vi "Main.vi"() -> ()   [LabVIEW 2014, in "Step Genie.lvlib"]
uses:
  Step Genie.lvlib
  <vilib>/Utility/error.llb/DialogType.ctl
  Source/SLL Queued State Machine/Queue Driver/Create Queue.vi
  Source/SLL Queued State Machine/Queue Driver/Enqueue an Item to Queue.vi
  Source/SLL Queued State Machine/Queue Driver/Dequeue Queue.vi
  Source/SLL Queued State Machine/Queue Driver/Enqueue N Items.vi
  Source/SLL Queued State Machine/Queue Driver/Flush Queue.vi
  Source/SLL Queued State Machine/Queue Driver/Release Queue.vi
  Source/SLL Queued State Machine/SLL QSM.lvlib
  Source/SLL Spreadsheet/SLL Spreadsheet.lvlib
panel:
  in  "Title":string(combo)
  in  "Fail":bool
  in  "Skip":bool
  in  "Pass":bool
  in  "Comments":string
  out "Instructions":string
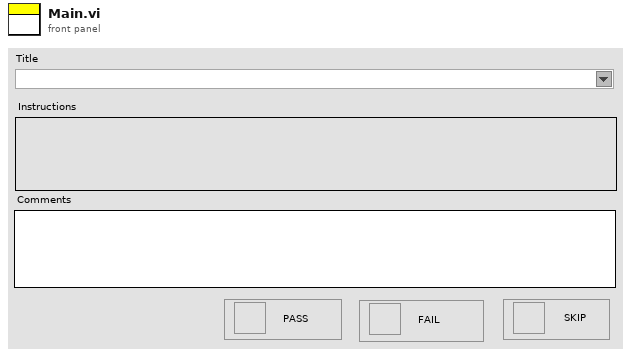
[diagram p1: front panel]
types:
  T1 = typedef "DialogType.ctl" = u16
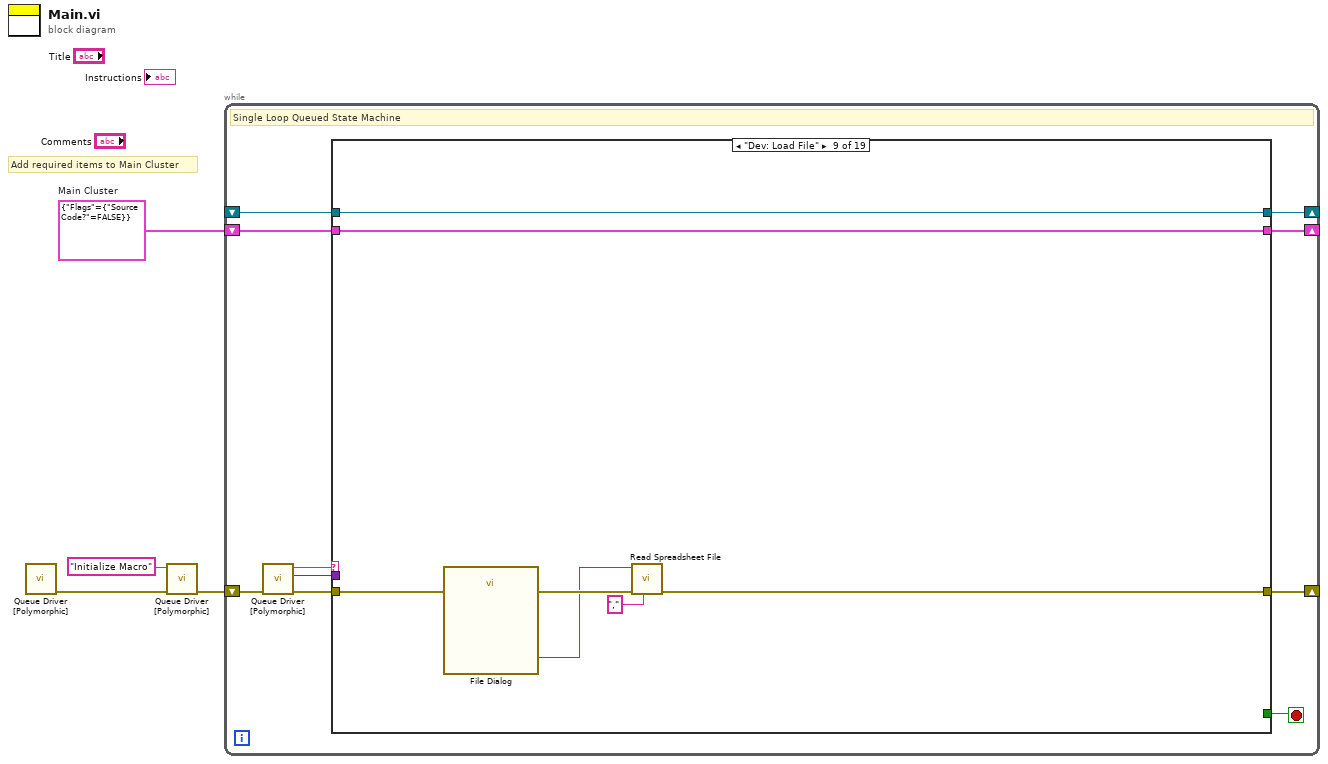
[diagram p0: block diagram]
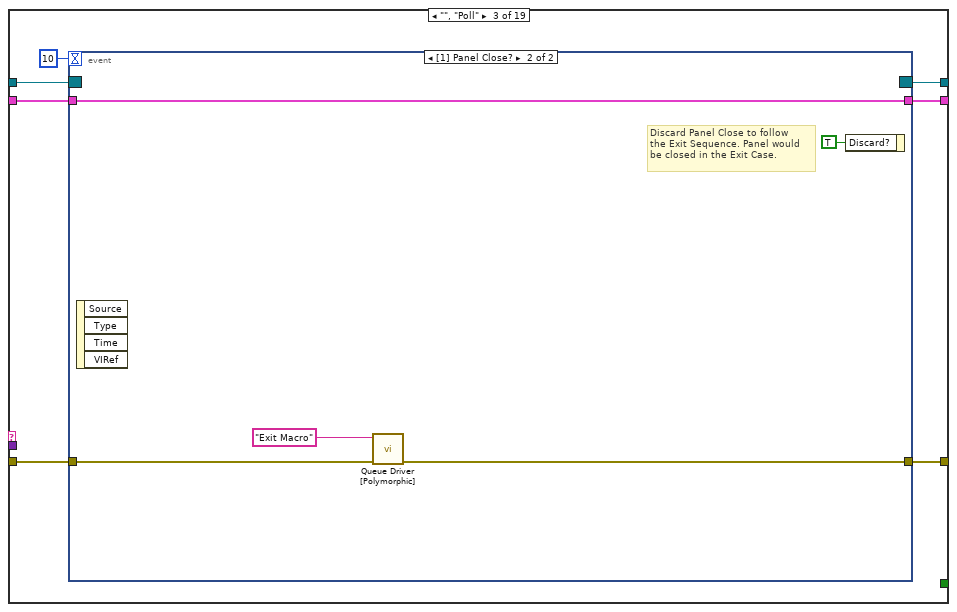
[diagram p4: hidden frame]
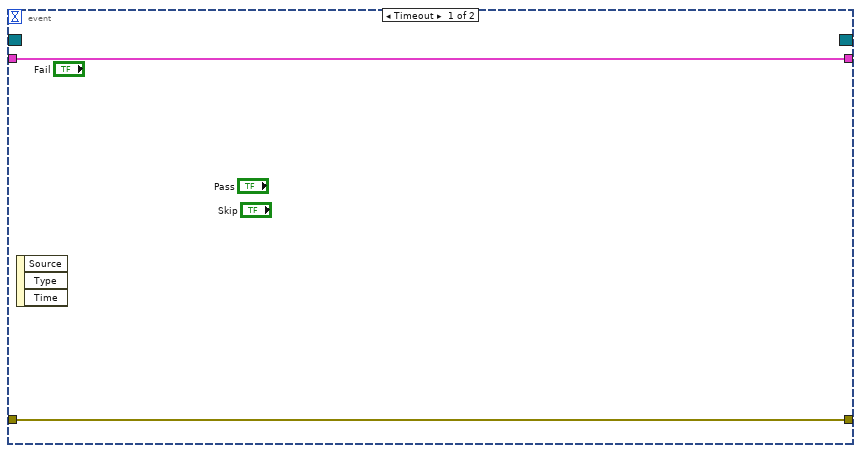
[diagram p5: hidden frame]
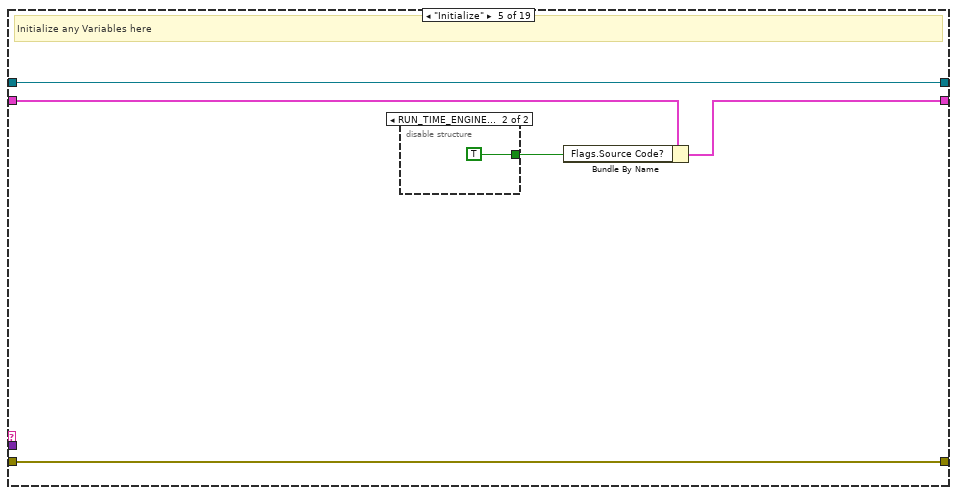
[diagram p7: hidden frame]
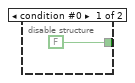
[diagram p8: hidden frame]
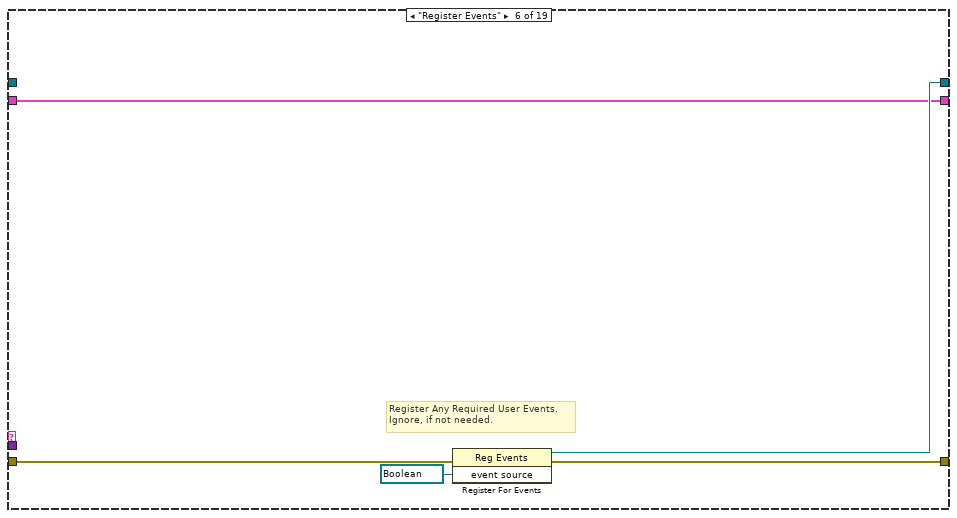
[diagram p9: hidden frame]
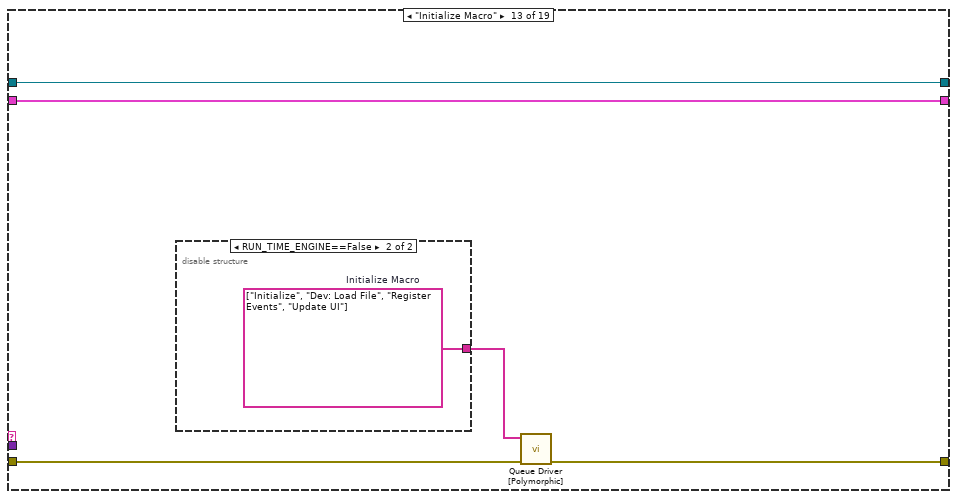
[diagram p15: hidden frame]
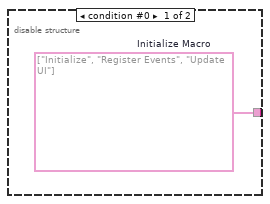
[diagram p16: hidden frame]
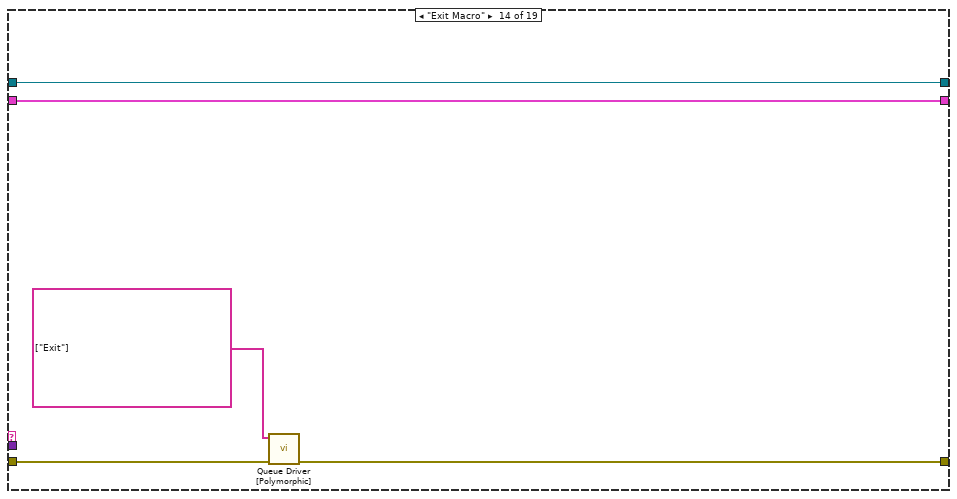
[diagram p17: hidden frame]
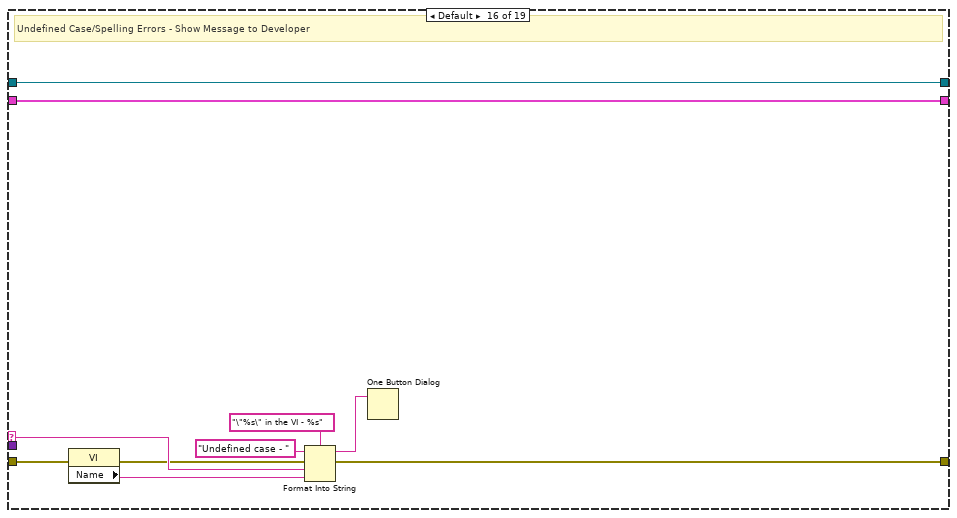
[diagram p19: hidden frame]
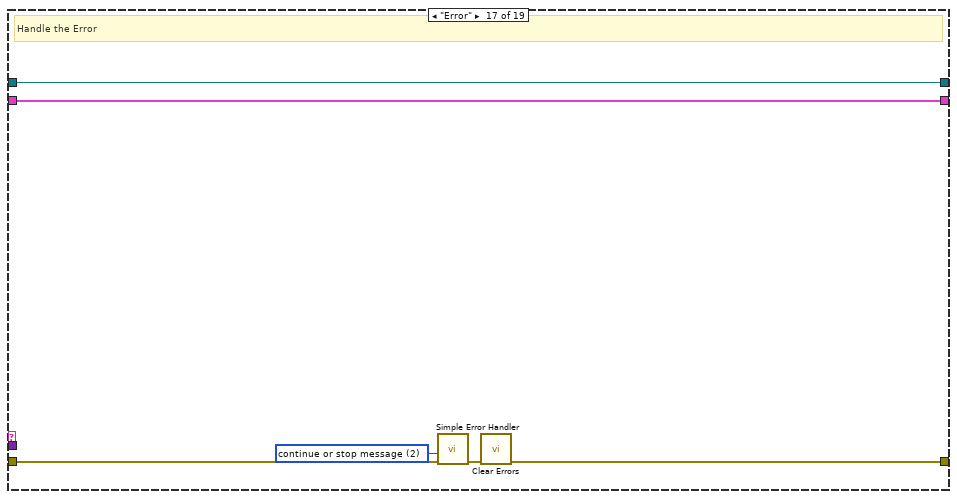
[diagram p20: hidden frame]
diagram:
  w3 = cluster{"Flags":cluster{"Source Code?":bool}} {"Flags"={"Source Code?"=FALSE}}  # Main Cluster
  # "Add required items to Main Cluster"
  n1 = call-poly "Queue Driver [Polymorphic].vi"() -> ("Error Out"=w1:errorcluster)  [unwired: 11 in]
  n2 = call-poly "Queue Driver [Polymorphic].vi"("Error In"=w1, "Item to Add"="Initialize Macro") -> ("Error Out"=w2:errorcluster)  [unwired: 9 in]
  n3 = while "SLL Queued State Machine" {
    shift-right: [w12] -> _
    shift-left: w2 -> [w14]
    shift-right: [w9] -> _
    shift-left: _ -> [w8]
    shift-right: [w7] -> _
    shift-left: w3 -> [w6]
    stop <- w11 stop-if-true
    # "Single Loop Queued State Machine"
    n4 = call-poly "Queue Driver [Polymorphic].vi"("Error In"=w14) -> ("Error Out"=w13:errorcluster, "Data"=w5:variant, "Dequeue"=w10:string)  [unwired: 8 in]
    n5 = case "QSM Case Structure" shown="\"Dev: Load File\"" w10 {
      selector: w10 -> [_ _ _ _ _ _ _ _ _ _ _ _ _ _ _ w90 _ _ _]
      tunnel: w13 -> [w17 w20 w25 w37 w42 w49 w52 w55 w62 w65 w68 w71 w74 w81 w86 w89 w102 w105 w116]
      tunnel: [w17 w20 w26 w37 w42 w48 w52 w55 w59 w65 w68 w71 w73 w80 w86 w93 w100 w105 w112] -> w12
      tunnel: [_ _ _ _ _ _ _ _ _ _ _ _ _ _ _ _ _ _ TRUE] -> w11
      tunnel: [w16 w19 w24 w36 w41 w47 w51 w54 w61 w64 w67 w70 w76 w83 w85 w96 w99 w104 w115] -> w9
      tunnel: w8 -> [w16 w19 w23 w36 w41 _ w51 w54 w61 w64 w67 w70 w76 w83 w85 w96 w99 w104 w115]
      tunnel: [w15 w18 w21 w35 w38 w46 w50 w53 w60 w63 w66 w69 w75 w82 w84 w95 w98 w103 w114] -> w7
      tunnel: w6 -> [w15 w18 w22 w35 w39 w46 w50 w53 w60 w63 w66 w69 w75 w82 w84 w95 w98 w103 w114]
      tunnel: w5 -> [_ _ _ _ _ _ _ _ _ _ _ _ _ _ _ _ _ _ _]
      frame "/--------------- Read Me -----------------/" {
        # "General Purpose Queue Based State Machine for Any Use Case (main application, module, pop up message etc)\n\nAdvantages:\n1. No Need to Pass Queue References between Queue Driver VIs.\n2. This template can be safely used in multiple parallel running modules without any issues.\n3. This template can also be safely used even in cases where the VI is configured to be a Clone, where multiple \ninstances of the VI could be executing concurrently.\n\nHow to Use:\n1. Add necessary items to the Main Cluster.\n2. Use the Polymorphic Queue Driver for doing any queue operations. There is no need to pass the queue driver\nreference, as the Queue Driver automatically infers the reference based on the VI instance from which it is called.\n3. Add any required user events in the \"Register Events\" case. Ignore if not needed.\n4. Use \"Sequences\" section for defining any list of state calls, which could be used in multiple places. \nEg: Initialize Sequence, might be needed if we need to any reinitialization."
      }
      frame "/------------------ Poll -------------------/" {
      }
      frame "", "Poll" {
        n6 = event shown="[1] Panel Close?" {
          selector: w23 -> [_ _]
          dyn-events: [_ _] -> w24
          timeout: 10 -> [_ _]
          tunnel: [w29 w33] -> w26
          tunnel: w25 -> [w29 w34]
          tunnel: w22 -> [w28 w32]
          tunnel: [w28 w32] -> w21
          event Timeout {
            n7 = event-data() -> ()  [unwired: 1 in, 3 out]
          }
          event Panel Close? {
            # "Discard Panel Close to follow\nthe Exit Sequence. Panel would\nbe closed in the Exit Case."
            n8 = event-data() -> ()  [unwired: 1 in, 4 out]
            n9 = call-poly "Queue Driver [Polymorphic].vi"("Error In"=w34, "Item to Add"="Exit Macro" ("Enqueue")) -> ("Error Out"=w33:errorcluster)  [unwired: 9 in]
            n10 = event-data("Discard?"=TRUE) -> ()  [unwired: 1 in, 1 out]
          }
        }
      }
      frame "/--------------- Initialize -----------------/" {
      }
      frame "Initialize" {
        # "Initialize any Variables here"
        n11 = disable-structure shown="RUN_TIME_ENGINE==False" {
          disable-tunnel: [FALSE TRUE] -> w40
          frame condition #0 {
          }
          frame condition #1 (active) {
          }
        }
        n12 = Bundle By Name(cluster=w39, "Flags.Source Code?"=w40) -> (w38:cluster{"Flags":cluster{"Source Code?":bool}})
      }
      frame "Register Events" {
        # "Register Any Required User Events. \nIgnore, if not needed."
        n13 = register-events(error in=w49, refnum<vi> refnum ("event source")) -> (reference out=w47:refnum<event-registration>, error out=w48:errorcluster)  [unwired: 1 in]
      }
      frame "/---------- Custom Case Splitter ----------/" {
      }
      frame "/----------------- Developer ---------------/" {
      }
      frame "Dev: Load File" {
        n14 = call "File Dialog"("error in"=w62) -> ("selected path"=w56:path, "error out"=w57:errorcluster)  [unwired: 11 in, 2 out]
        n15 = call "Read Spreadsheet File.vi"("Delimiter (tab)"=",", "error in (no error)"=w57, "File Path"=w56) -> ("error out"=w59:errorcluster)  [unwired: 7 in, 1 out]
      }
      frame "/-------------- User Interface --------------/" {
        # "Duplicate this case to create additional case splitters for readability"
      }
      frame "Update UI" {
        # "Update Front Panel Controls in this Case"
      }
      frame "/----------------- Macros -----------------/" {
      }
      frame "Initialize Macro" {
        n16 = disable-structure shown="RUN_TIME_ENGINE==False" {
          disable-tunnel: [w77 w78] -> w72
          frame condition #0 {
            w77 = string[] ["Initialize", "Register Events", "Update UI"]  # Initialize Macro
          }
          frame condition #1 (active) {
            w78 = string[] ["Initialize", "Dev: Load File", "Register Events", "Update UI"]  # Initialize Macro
          }
        }
        n17 = call-poly "Queue Driver [Polymorphic].vi"("Error In"=w74, "Enqueue N"=w72) -> ("Error Out"=w73:errorcluster)  [unwired: 9 in]
      }
      frame "Exit Macro" {
        n18 = call-poly "Queue Driver [Polymorphic].vi"("Error In"=w81, "Enqueue N"=string[] ["Exit"]) -> ("Error Out"=w80:errorcluster)  [unwired: 9 in]
      }
      frame "/-------------- Error Handler--------------/" {
      }
      frame Default {
        # "Undefined Case/Spelling Errors - Show Message to Developer"
        n19 = property class="VI"(error in=w89) -> (error out=w88:errorcluster, "Name"=w87:string)  [unwired: 1 in, 1 out]
        n20 = Format Into String(format string="\"%s\" in the VI - %s" ("message"), initial string="Undefined case - ", error in=w88, w90, w87) -> (resulting string=w91:string, error out=w93:errorcluster)
        n21 = One Button Dialog(message=w91) -> ()  [unwired: 1 in, 1 out]
      }
      frame "Error" {
        w97 = T1 2 items=["no dialog", "OK message", "continue or stop message", "OK message + warnings", "continue/stop + warnings"] ("type of dialog (OK msg:1)")
        # "Handle the Error"
        n22 = call <vilib>:"Simple Error Handler.vi"("type of dialog (OK msg:1)"=w97, "error in (no error)"=w102) -> ("error out"=w101:errorcluster)  [unwired: 3 in, 4 out]
        n23 = call <vilib>:"Clear Errors.vi"("error in (no error)"=w101) -> ("error out"=w100:errorcluster)  [unwired: 5 in, 1 out]
      }
      frame "/------------------- Exit --------------------/" {
      }
      frame "Exit" {
        n24 = call-poly "Queue Driver [Polymorphic].vi"("Error In"=w116) -> ("Error Out"=w117:errorcluster)  [unwired: 9 in, 1 out]
        n25 = Unbundle By Name(w114) -> ("Flags.Source Code?"=w107:bool)
        n26 = call-poly "Queue Driver [Polymorphic].vi"("Error In"=w117) -> ("Error Out"=w113:errorcluster)  [unwired: 10 in]
        n27 = Call Chain() -> (call chain=w111:string[])
        n28 = Array Size(array=w111) -> (size(s)=w110:i32)
        n29 = Equal?(x=w110, y=1) -> (x = y?=w108:bool)
        n30 = And(x=w107, y=w108) -> (x .and. y?=w106:bool)
        n31 = case "Skip Panel Close when in Source\nCode and is the top most caller" shown="False" w106 {
          tunnel: w113 -> [w120 w122]
          tunnel: [w121 w122] -> w112
          frame False {
            # "Close Panel"
            n32 = invoke class="VI" method="FP.Close"() -> (error out=w119:errorcluster)  [unwired: 3 in, 2 out]
            n33 = Merge Errors(w120, w119) -> (w121:errorcluster)
          }
          frame True {
            # "Do Not Close Panel"
          }
        }
      }
    }
  }
